vi "Parse Structure Recursive with Fast Tree--Replacement.vi"(8 "error in":errorcluster, 10 "Node":T1, 11 "ParseGDSII in":refnum<class "ParseGDSII.lvclass">) -> (0 "error out":errorcluster, 2 "Geometric Objects":refnum<class "Geometric.lvclass">[](array[class]), 3 "ParseGDSII out":refnum<class "ParseGDSII.lvclass">)   [LabVIEW 2019, in "ParseGDSII.lvclass"]
uses:
  ParseGDSII.lvclass
  Elements/Geometric.lvclass
  C:/Users/Albro/Documents/GitHub/AFM-Lithography/lvsrc/Classes/Parse/GDSII/Elements/Element.lvclass
  Elements/Referential.lvclass
  Elements/Element.lvclass
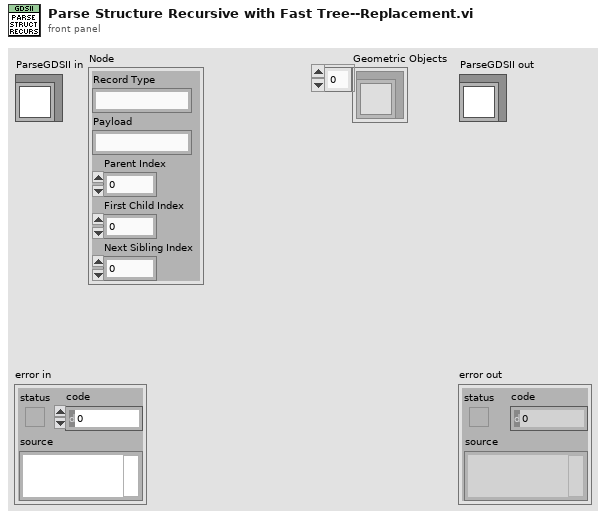
[diagram p1: front panel]
types:
  T1 = cluster{"Record Type":string, "Payload":string, "Parent Index":i32, "First Child Index":i32, "Next Sibling Index":i32}
  T2 = cluster{"Record Type":string, "Payload":string, "Parent Index":i32, "First Child Index":i32, "Next Sibling Index":i32}[]
  T3 = typedef "NI_Matrix.lvlib/RealMatrix.ctl" = dbl[][]
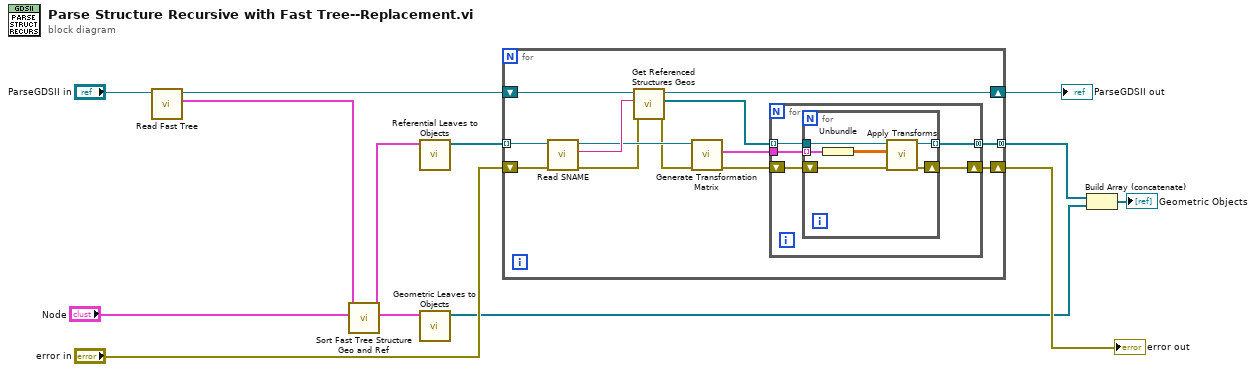
[diagram p0: block diagram]
diagram:
  n1 = call "Read Fast Tree.vi"("ParseGDSII in"="ParseGDSII in") -> ("Tree"=w11:T2, "ParseGDSII out"=w9:refnum<class "ParseGDSII.lvclass">)  [unwired: 7 in, 2 out]
  n2 = call "Sort Fast Tree Structure Geo and Ref.vi"("Node"="Node", "Tree"=w11) -> ("Geometric Items"=w4:T2, "Reference Items"=w10:T2)  [unwired: 8 in]
  n3 = call "Referential Leaves to Objects.vi"("Reference Items"=w10) -> ("Reference Objects"=w8:refnum<class "Referential.lvclass">[])  [unwired: 10 in]
  n4 = call "Geometric Leaves to Objects.vi"("Geometric Items"=w4) -> ("Geometric Objects"=w2:refnum<class "Geometric.lvclass">[])  [unwired: 10 in]
  n5 = for {
    shift-right: [w24] -> w5
    shift-left: w9 -> [w25]
    tunnel: w8 -> [w26] mode=indexing
    shift-right: [w15] -> w6
    shift-left: "error in" -> [w19]
    tunnel: [w14] -> w3 mode=concatenating
    n6 = call-dynamic "Read SNAME.vi"("error in (no error)"=w19, "Referential in"=w26) -> ("error out"=w21:errorcluster, "SNAME"=w23:string, "Referential out"=w22:refnum<class "Referential.lvclass">)  [unwired: 7 in]
    n7 = call "Get Referenced Structures Geos.vi"("error in"=w21, "SNAME"=w23, "ParseGDSII in"=w25) -> ("error out"=w20:errorcluster, "Geometric"=w17:refnum<class "Geometric.lvclass">[], "ParseGDSII out"=w24:refnum<class "ParseGDSII.lvclass">)  [unwired: 6 in]
    n8 = call "Generate Transformation Matrix.vi"("error in"=w20, "Referential in"=w22) -> ("error out"=w16:errorcluster, "Matrix Array"=w18:cluster{"A x B":T3}[])  [unwired: 7 in, 1 out]
    n9 = for {
      tunnel: w17 -> [w31] mode=indexing
      tunnel: w18 -> [w30]
      shift-right: [w28] -> w15
      shift-left: w16 -> [w29]
      tunnel: [w27] -> w14 mode=concatenating
      n10 = for {
        tunnel: w31 -> [w37]
        tunnel: w30 -> [w36] mode=indexing
        shift-right: [w33] -> w28
        shift-left: w29 -> [w34]
        tunnel: [w32] -> w27 mode=indexing
        n11 = Unbundle(w36) -> ("A x B"=w35:T3)
        n12 = call "Apply Transforms.vi"("error in"=w34, "Matrix"=w35, "Element in"=w37) -> ("error out"=w33:errorcluster, "Element out"=w32:refnum<class "Geometric.lvclass">)  [unwired: 7 in]
      }
    }
  }
  "error out" <- w6
  "ParseGDSII out" <- w5
  n13 = Build Array (concatenate)(w3, w2) -> (→"Geometric Objects":refnum<class "Geometric.lvclass">[])
